vi "Lockin.DAQ.Configure Sweep.vi"(8 "error in (no error)":errorcluster, 11 "Lockin.DAQ in":refnum<class "Lockin.DAQ.lvclass">) -> (0 "error out":errorcluster, 3 "Lockin.DAQ out":refnum<class "Lockin.DAQ.lvclass">)   [LabVIEW 2016, in "Lockin.DAQ.lvclass"]
uses:
  Lockin.DAQ.lvclass
  Lockin.DAQ.lvclass/Lockin.DAQ.ctl
  Typedefs/Function-enum.ctl
panel:
  out "Frequency (Hz)":dbl
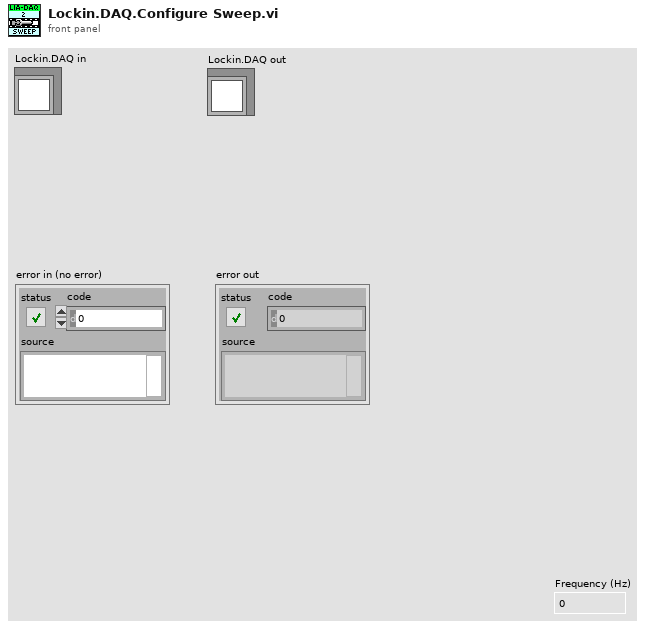
[diagram p1: front panel]
types:
  T1 = typedef "Lockin.DAQ.lvclass/AO-cluster.ctl" = cluster{"Ch":i32[], "Amp (V)":dbl[], "DC (V)":dbl[], "f (Hz)":dbl[], "Phase (°)":dbl[], "Function":T2[], "Sweep?":bool[]}
  T2 = typedef "Lockin.DAQ.lvclass/Function-enum.ctl" = enum16{"Sine", "Triangle", "Square", "Sawtooth"}
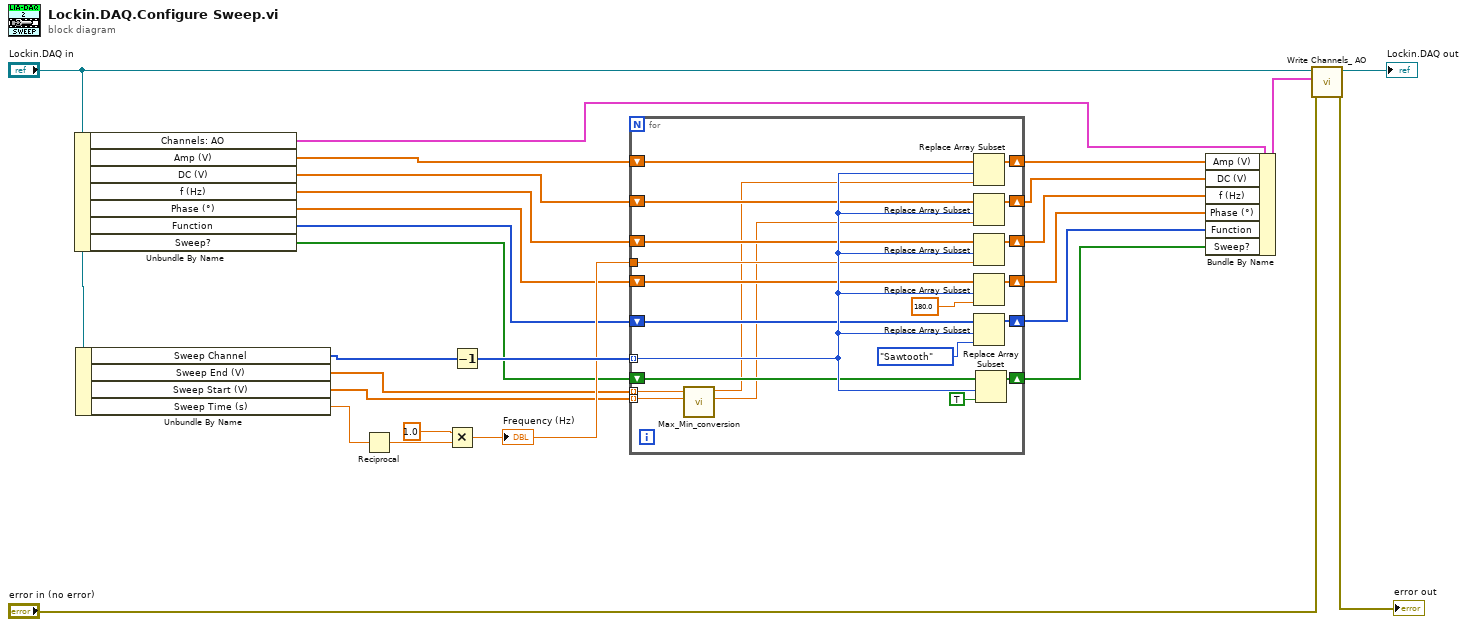
[diagram p0: block diagram]
diagram:
  n1 = Unbundle By Name("Lockin.DAQ in") -> ("Channels: AO"=w1:T1, "Amp (V)"=w18:dbl[], "DC (V)"=w17:dbl[], "f (Hz)"=w16:dbl[], "Phase (°)"=w15:dbl[], "Function"=w14:T2[], "Sweep?"=w13:bool[])
  n2 = Unbundle By Name("Lockin.DAQ in") -> ("Sweep Channel"=w6:i32[], "Sweep End (V)"=w3:dbl[], "Sweep Start (V)"=w2:dbl[], "Sweep Time (s)"=w4:dbl)
  n3 = Reciprocal(x=w4) -> (1/x=w22:dbl)
  n4 = Multiply(x=1.0, y=w22) -> (x*y=w20:dbl)
  "Frequency (Hz)" <- w20
  n5 = Decrement(x=w6) -> (x-1=w21:i32[])
  n6 = for {
    tunnel: w21 -> [w44] mode=indexing
    tunnel: w20 -> [w43]
    shift-right: [w36] -> w12
    shift-left: w18 -> [w42]
    shift-right: [w35] -> w11
    shift-left: w17 -> [w41]
    shift-right: [w34] -> w10
    shift-left: w16 -> [w40]
    shift-right: [w33] -> w9
    shift-left: w15 -> [w39]
    shift-right: [w32] -> w8
    shift-left: w14 -> [w38]
    shift-right: [w31] -> w7
    shift-left: w13 -> [w37]
    tunnel: w3 -> [w28] mode=indexing
    tunnel: w2 -> [w27] mode=indexing
    n7 = call <userlib>:"Max_Min_conversion.vi"("Min"=w27, "Max"=w28) -> ("offset"=w29:dbl, "Amplitude"=w30:dbl)  [unwired: 8 in]
    n8 = Replace Array Subset(array=w42, new element=w30, index=w44) -> (w36:dbl[])
    n9 = Replace Array Subset(array=w41, new element=w29, index=w44) -> (w35:dbl[])
    n10 = Replace Array Subset(array=w40, new element=w43, index=w44) -> (w34:dbl[])
    n11 = Replace Array Subset(array=w39, new element=180.0 ("new element/subarray"), index=w44) -> (w33:dbl[])
    n12 = Replace Array Subset(array=w38, new element=Function-enum."Sawtooth" ("new element/subarray"), index=w44) -> (w32:T2[])
    n13 = Replace Array Subset(array=w37, new element=TRUE ("new element/subarray"), index=w44) -> (w31:bool[])
  }
  n14 = Bundle By Name(cluster=w1, "Amp (V)"=w12, "DC (V)"=w11, "f (Hz)"=w10, "Phase (°)"=w9, "Function"=w8, "Sweep?"=w7) -> (w23:T1)
  n15 = call "Write Channels_ AO.vi"("error in (no error)"="error in (no error)", "Channels: AO"=w23, "Lockin.DAQ"="Lockin.DAQ in") -> ("error out"=→"error out":errorcluster, "Lockin.DAQ out"=→"Lockin.DAQ out":refnum<class "Lockin.DAQ.lvclass">)  [unwired: 7 in]
